vi "I16toI15.vi"(0 "Array":u16[](array[numeric]) format="%.6f") -> (1 "logical AND":bool, 2 "Array 2":i16[](array[numeric]))   [LabVIEW 2016]
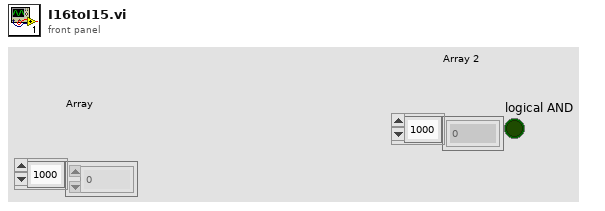
[diagram p1: front panel]
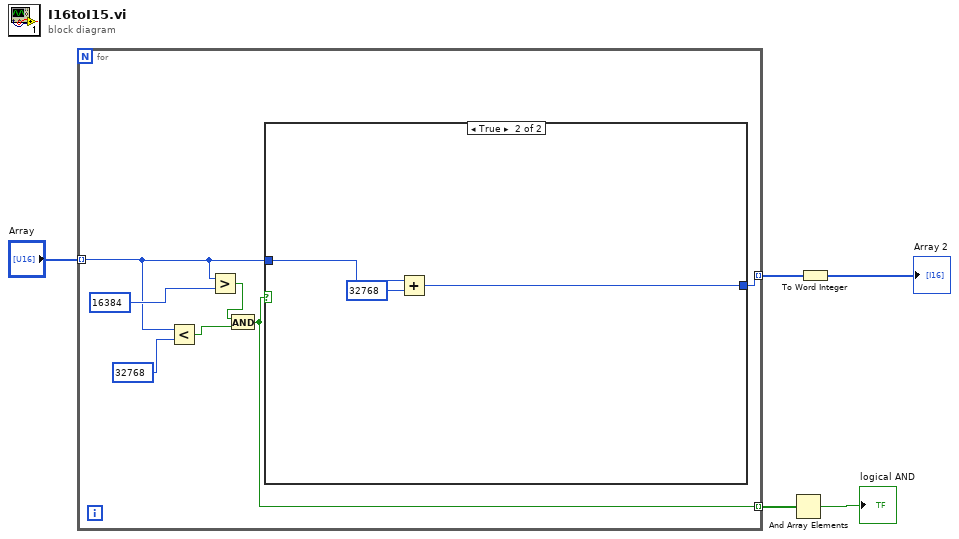
[diagram p0: block diagram]
diagram:
  n1 = for {
    tunnel: "Array" -> [w9] mode=indexing
    tunnel: [w11] -> w4 mode=indexing
    tunnel: [w6] -> w2 mode=indexing
    n2 = Less?(x=w9, y=u16 32768) -> (x < y?=w8:bool)
    n3 = Greater?(x=w9, y=u16 16384) -> (0:w10:bool)
    n4 = And(x=w10, y=w8) -> (x .and. y?=w6:bool)
    n5 = case shown="True" w6 {
      tunnel: w9 -> [w13 w16]
      tunnel: [w13 w14] -> w11
      frame False {
      }
      frame True {
        n6 = Add(x=w16, y=u16 32768) -> (x+y=w14:u16)
      }
    }
  }
  n7 = And Array Elements(Boolean array=w2) -> (logical AND=→"logical AND":bool)
  n8 = To Word Integer(number=w4) -> (16bit integer=→"Array 2":i16[])
